vi "ConverteixAsg.vi"(11 "Value":dbl) -> (3 "Numeric":i32)   [LabVIEW 2017]
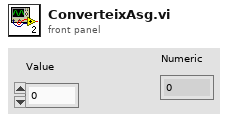
[diagram p1: front panel]
types:
  T1 = typedef "LVDateTimeRec.ctl" = cluster{"fractional second":dbl, "second":i32, "minute":i32, "hour":i32, "day of month":i32, "month":i32, "year":i32, "day of week":i32, "day of year":i32, "DST":i32}
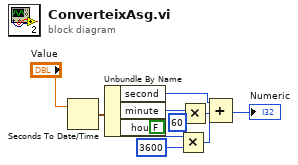
[diagram p0: block diagram]
diagram:
  (unwired) FALSE
  n1 = Seconds To Date/Time(time stamp (now)="Value") -> (date time rec=w2:T1)  [unwired: 1 in]
  n2 = Unbundle By Name(w2) -> ("second"=w8:i32, "minute"=w5:i32, "hour"=w3:i32)
  n3 = Multiply(x=w3, y=3600) -> (x*y=w9:i32)
  n4 = Multiply(x=w5, y=60) -> (x*y=w7:i32)
  n5 = Compound Arithmetic op=ADD(w8, w7, w9) -> (→"Numeric":i32)
